vi "Initialise Picture.vi"(8 "error in (no error)":errorcluster, 10 "picture":picture) -> (0 "error out":errorcluster, 1 "Valid":bool, 3 "Grassfire 2D out":refnum<class "Grassfire 2D.lvclass">)   [LabVIEW 2019, in "Grassfire 2D.lvclass"]
uses:
  Grassfire 2D.lvclass
  Node Address--cluster.ctl
  Node Value--cluster.ctl
  Shared/Node Type--enum.ctl
  Grassfire 2D.lvclass/Grassfire 2D.ctl
  Shared/Shared.lvlib
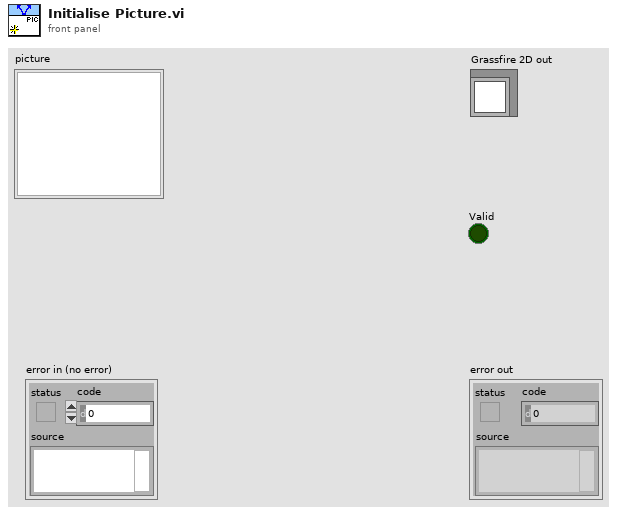
[diagram p1: front panel]
types:
  T1 = typedef "imagedata.ctl" = cluster{"image type":i32, "image depth":i32, "image":u8[], "mask":u8[], "colors":u32[], "Rectangle":cluster{"left":i16, "top":i16, "right":i16, "bottom":i16}}
  T2 = typedef "Grassfire 2D.lvclass/Node Address--cluster.ctl" = cluster{"Row":i32, "Column":i32}
  T3 = typedef "Grassfire 2D.lvclass/Node Value--cluster.ctl" = cluster{"Type":T4, "Distance":i32}
  T4 = typedef "Shared.lvlib/Node Type--enum.ctl" = enum16{"Empty", "Blocked", "Start", "End", "Path"}
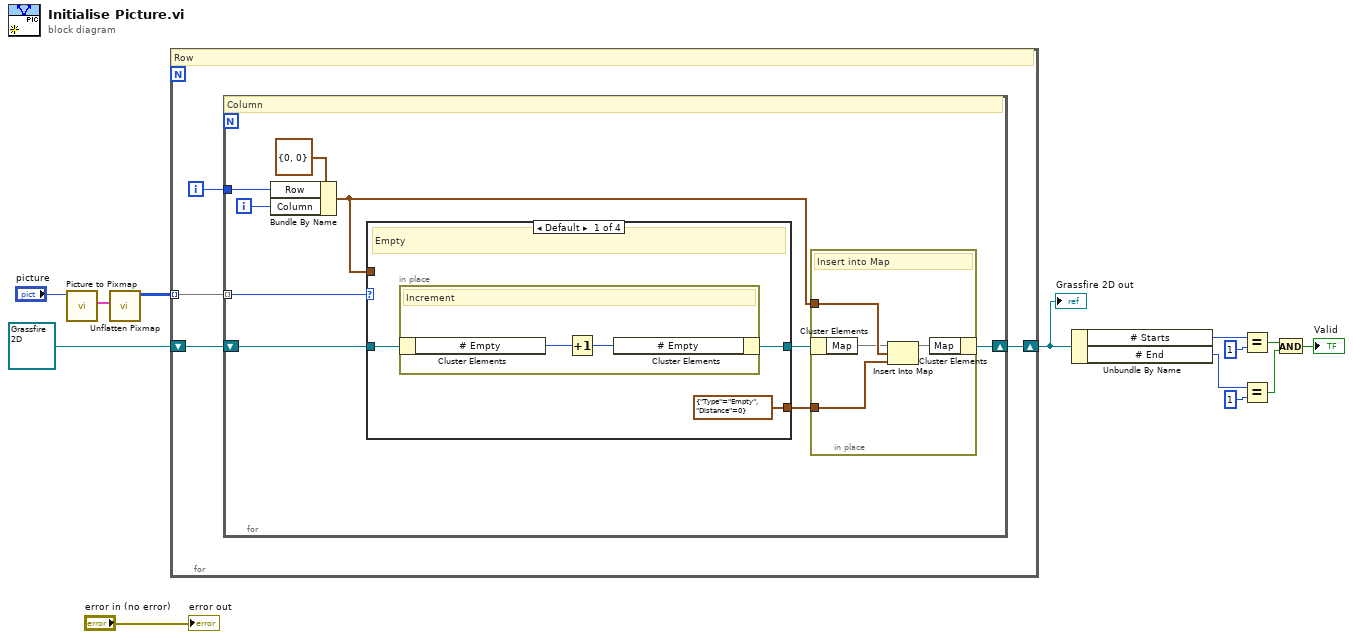
[diagram p0: block diagram]
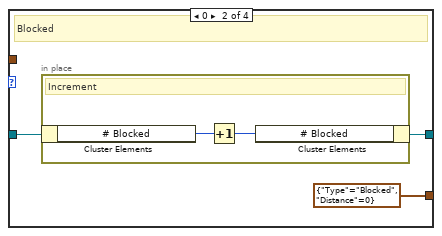
[diagram p2: hidden frame]
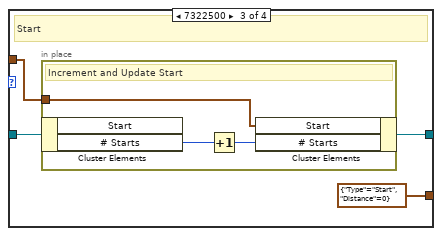
[diagram p3: hidden frame]
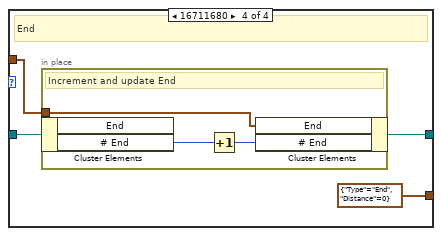
[diagram p4: hidden frame]
diagram:
  n1 = call <vilib>:"Picture to Pixmap.vi"("picture"="picture") -> ("image data"=w3:T1)  [unwired: 9 in, 1 out]
  n2 = call <vilib>:"Unflatten Pixmap.vi"("image data"=w3) -> ("24-bit pixmap"=w2:u32[][])  [unwired: 4 in, 6 out]
  n3 = for {
    shift-right: [w16] -> w5
    shift-left: refnum<class "Grassfire 2D.lvclass"> refnum ("Grassfire 2D out") -> [w17]
    tunnel: w2 -> [w14] mode=indexing
    i -> [w15]
    # "Row"
    n4 = for {
      shift-right: [w24] -> w16
      shift-left: w17 -> [w26]
      tunnel: w15 -> [w22]
      tunnel: w14 -> [w18] mode=indexing
      i -> [w21]
      # "Column"
      n5 = Bundle By Name(cluster=T2 {"Row"=0, "Column"=0} ("Address"), "Row"=w22, "Column"=w21) -> (w19:T2)
      n6 = case shown="Default" w18 {
        tunnel: w26 -> [w33 w38 w44 w51]
        tunnel: [w32 w37 w43 w50] -> w25
        tunnel: [T3 {"Type"=enum."Empty", "Distance"=0} ("Value") T3 {"Type"=enum."Blocked", "Distance"=0} ("Value") T3 {"Type"=enum."Start", "Distance"=0} ("Value") T3 {"Type"=enum."End", "Distance"=0} ("Value")] -> w20
        tunnel: w19 -> [_ _ w41 w49]
        frame Default {
          # "Empty"
          n7 = in-place {
            # "Increment"
            n8 = in-place-cluster #1(w33) -> ("# Empty"=w35:i32)
            n9 = Increment(x=w35) -> (x+1=w34:i32)
            n10 = in-place-cluster #1("# Empty"=w34) -> (w32:refnum<class "Grassfire 2D.lvclass">)
          }
        }
        frame 0 {
          # "Blocked"
          n11 = in-place {
            # "Increment"
            n12 = in-place-cluster #2(w38) -> ("# Blocked"=w40:i32)
            n13 = Increment(x=w40) -> (x+1=w39:i32)
            n14 = in-place-cluster #2("# Blocked"=w39) -> (w37:refnum<class "Grassfire 2D.lvclass">)
          }
        }
        frame 7322500 {
          # "Start"
          n15 = in-place {
            in-place-border: w41 -> [w45]
            # "Increment and Update Start"
            n16 = in-place-cluster #3(w44) -> ("# Starts"=w47:i32)  [unwired: 1 out]
            n17 = Increment(x=w47) -> (x+1=w46:i32)
            n18 = in-place-cluster #3("Start"=w45, "# Starts"=w46) -> (w43:refnum<class "Grassfire 2D.lvclass">)
          }
        }
        frame 16711680 {
          # "End"
          n19 = in-place {
            in-place-border: w49 -> [w52]
            # "Increment and update End"
            n20 = in-place-cluster #4(w51) -> ("# End"=w54:i32)  [unwired: 1 out]
            n21 = Increment(x=w54) -> (x+1=w53:i32)
            n22 = in-place-cluster #4("End"=w52, "# End"=w53) -> (w50:refnum<class "Grassfire 2D.lvclass">)
          }
        }
      }
      n23 = in-place {
        in-place-border: w19 -> [w28]
        in-place-border: w20 -> [w29]
        # "Insert into Map"
        n24 = in-place-cluster #5(w25) -> ("Map"=w27:map{T2, T3})
        n25 = Insert Into Map(map in=w27, key=w28, value=w29) -> (map out=w30:map{T2, T3})  [unwired: 2 out]
        n26 = in-place-cluster #5("Map"=w30) -> (w24:refnum<class "Grassfire 2D.lvclass">)
      }
    }
  }
  "Grassfire 2D out" <- w5
  n27 = Unbundle By Name(w5) -> ("# Starts"=w12:i32, "# End"=w13:i32)
  n28 = Equal?(x=w12, y=1) -> (x = y?=w9:bool)
  n29 = Equal?(x=w13, y=1) -> (x = y?=w11:bool)
  n30 = And(x=w9, y=w11) -> (x .and. y?=→"Valid":bool)
  "error out" <- "error in (no error)"
